vi "Get Radio Button Text and Label.vi"(0 "error in":refnum<vi>, 11 "filenames in":errorcluster) -> (4 "selected Buton.Text":string, 6 "selected Label.Text":string, 8 "Button.Text []":string[](array[string]), 10 "Label.Text []":string[](array[string]), 15 "filenames out":errorcluster)   [LabVIEW 2019]
doc: "Get Text and Label from Radio Button."
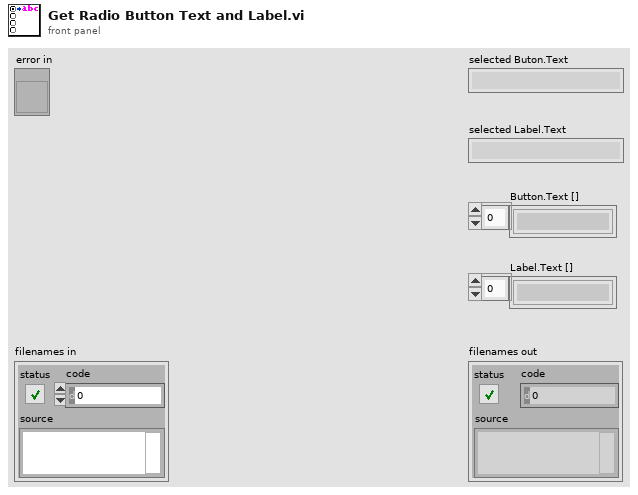
[diagram p1: front panel]
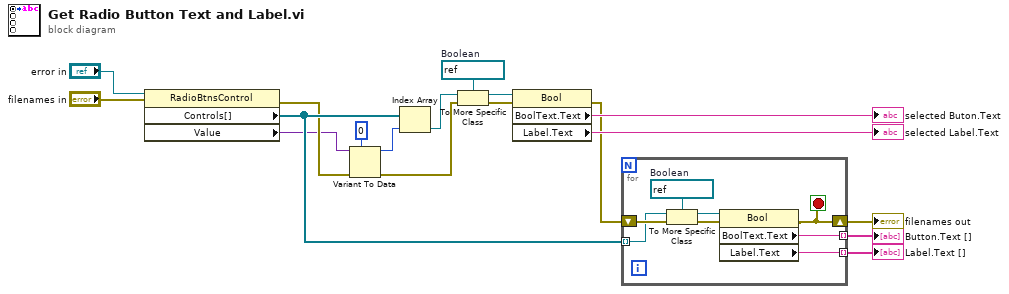
[diagram p0: block diagram]
diagram:
  w17 = refnum<vi> refnum  # Boolean
  n1 = property class="RadioBtnsControl"(reference="error in", error in="filenames in") -> (error out=w5:errorcluster, "Controls[]"=w10:refnum<vi>[], "Value"=w3:variant)  [unwired: 1 out]
  n2 = Variant To Data(error in=w5, type=u32 0, Variant=w3) -> (data=w2:u32, error out=w4:errorcluster)
  n3 = Index Array(array=w10, index=w2) -> (element=w15:refnum<vi>)
  n4 = To More Specific Class(target class=w17, reference=w15, error in=w4) -> (specific class reference=w16:refnum<vi>, error out=w18:errorcluster)
  n5 = property class="Bool"(reference=w16, error in=w18) -> (error out=w8:errorcluster, "BoolText.Text"=→"selected Buton.Text":string, "Label.Text"=→"selected Label.Text":string)  [unwired: 1 out]
  n6 = for {
    tunnel: w10 -> [w21] mode=indexing
    shift-right: [w22] -> w9
    shift-left: w8 -> [w25]
    tunnel: [w20] -> w7 mode=indexing
    tunnel: [w19] -> w6 mode=indexing
    stop <- w22 stop-if-true
    w26 = refnum<vi> refnum  # Boolean
    n7 = To More Specific Class(target class=w26, reference=w21, error in=w25) -> (specific class reference=w24:refnum<vi>, error out=w23:errorcluster)
    n8 = property class="Bool"(reference=w24, error in=w23) -> (error out=w22:errorcluster, "BoolText.Text"=w20:string, "Label.Text"=w19:string)  [unwired: 1 out]
  }
  "filenames out" <- w9
  "Button.Text []" <- w7
  "Label.Text []" <- w6
